vi "Output Enable Read Array.vi"(8 "error in":errorcluster, 9 "Number of Channels":u32=1, 11 "Output Enable in":refnum<class "Output Enable.lvclass">) -> (0 "error out":errorcluster, 1 "Changed or First Call?":bool, 2 "Current Output":bool[](array[boolean]), 3 "Output Enable out":refnum<class "Output Enable.lvclass">)   [LabVIEW 2023, in "Output Enable.lvclass"]
uses:
  Output Enable.lvclass
  Output Enable.lvclass/Output Enable.ctl
  <vilib>/ADAS Replay HIL/Channels/Tag Wrapper/Polymorphic/Read Channel (Boolean).vi
  693d6ef1-dc9b-43af-acaf-871d9c3806ee.vi
  <vilib>/ADAS Replay HIL/Channels/Tag Wrapper/Polymorphic/Read Channel (Boolean).vi/b2f764de-0c1e-4784-a155-687fc995a684.vi
  <vilib>/ADAS Replay HIL/Channels/Tag Wrapper/Polymorphic/Read Channel (Boolean).vi/b2f764de-0c1e-4784-a155-687fc995a684.vi/c28b0ead-42ad-4072-80a2-aca7f2bd7ce3.vi
  <vilib>/ADAS Replay HIL/Channels/Tag Wrapper/Polymorphic/Read Channel (Boolean).vi/b2f764de-0c1e-4784-a155-687fc995a684.vi/219d0231-d98b-4193-b5cc-84f90e3c9091.vi
  <vilib>/ADAS Replay HIL/Channels/Tag Wrapper/Tag Wrapper.lvlib
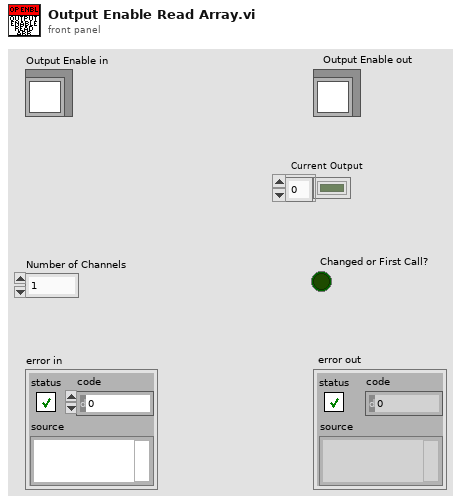
[diagram p1: front panel]
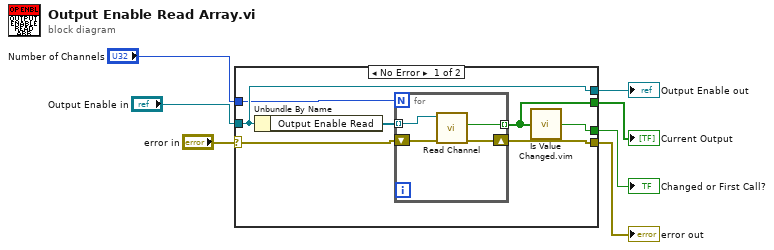
[diagram p0: block diagram]
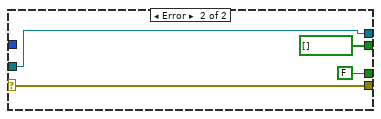
[diagram p2: hidden frame]
diagram:
  n1 = case shown="No Error" "error in" {
    selector: "error in" -> [w14 w22]
    tunnel: [w13 w22] -> w6
    tunnel: [w9 w21] -> w3
    tunnel: "Output Enable in" -> [w9 w21]
    tunnel: [w12 bool[] []] -> w2
    tunnel: [w11 FALSE ("changed or first call?")] -> w5
    tunnel: "Number of Channels" -> [w8 _]
    frame No Error {
      n2 = Unbundle By Name(w9) -> ("Output Enable Read"=w10:refnum<k21>[])
      n3 = for {
        N: w8 -> [_]
        tunnel: [w16] -> w12 mode=indexing
        shift-right: [w17] -> w13
        shift-left: w14 -> [w18]
        tunnel: w10 -> [w15] mode=indexing
        n4 = call-poly <vilib>:"Read Channel.vi"("error in"=w18, "ADAS HIL Channel in"=w15) -> ("error out"=w17:errorcluster, "Value out"=w16:bool)  [unwired: 6 in, 2 out]
      }
      n5 = call "Is Value Changed.vim"("value"=w12) -> ("changed or first call?"=w11:bool)
    }
    frame Error {
    }
  }
  "error out" <- w6
  "Changed or First Call?" <- w5
  "Output Enable out" <- w3
  "Current Output" <- w2
